vi "Processed_Bytes_To_Data_Packet.vi"(2 "Processed Bytes":u8[](array[numeric]), 3 "Data Packet In":T1) -> (1 "Data Packet Out":T1)   [LabVIEW 2017]
uses:
  Controls/Packet/Packet.ctl
  Controls/Packet/Packet_Direction.ctl
  Controls/Packet/Packet_Type.ctl
  Controls/Packet/Packet_Priority.ctl
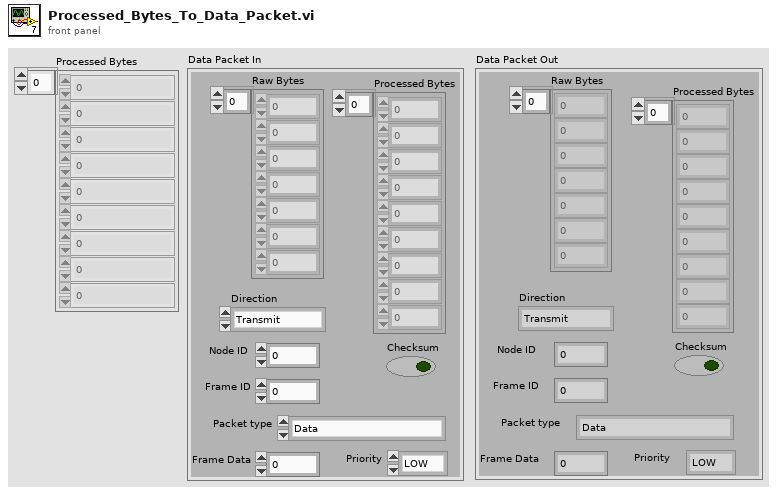
[diagram p1: front panel]
types:
  T1 = typedef "Packet.ctl" = cluster{"Raw Bytes":u8[], "Checksum":bool, "Direction":T2, "Processed Bytes":u8[], "Node ID":u8, "Packet type":T3, "Frame Data":u32, "Priority":T4, "Frame ID":u8}
  T2 = typedef "Packet_Direction.ctl" = enum16{"Transmit", "Receive", "Bidirectional"}
  T3 = typedef "Packet_Type.ctl" = enum16{"Data", "Connection Management", "Remote Request", "Error/Status"}
  T4 = typedef "Packet_Priority.ctl" = enum16{"LOW", "HIGH"}
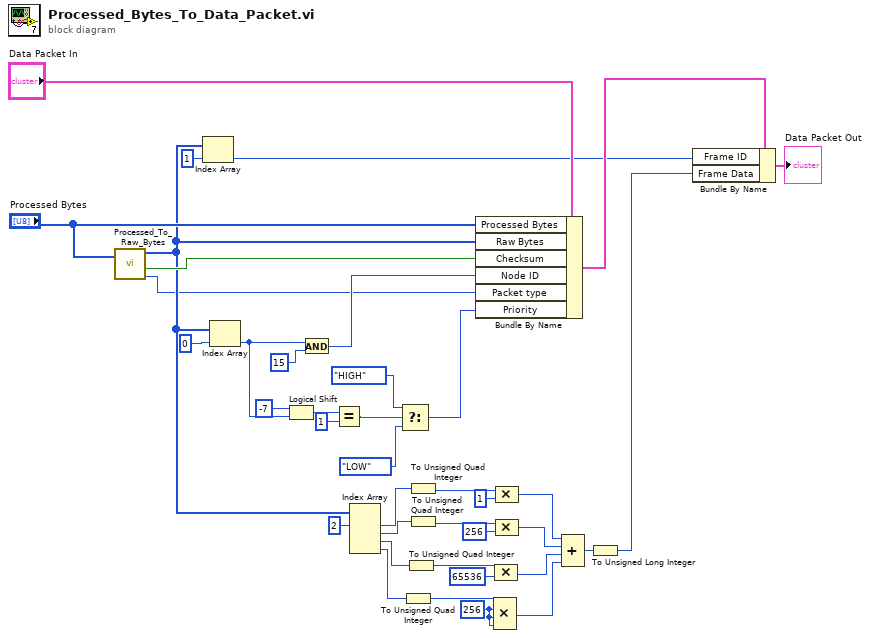
[diagram p0: block diagram]
diagram:
  w9 = u64 256 ("value")
  n1 = call "Processed_To_Raw_Bytes.vi"("Processed Bytes"="Processed Bytes") -> ("Packet Type"=w1:T3, "Checksum"=w37:bool, "Raw Bytes"=w22:u8[])  [unwired: 1 in, 2 out]
  n2 = Index Array(array=w22, index=1) -> (element=w23:u8)
  n3 = Index Array(array=w22, index=0) -> (element=w33:u8)
  n4 = Logical Shift(y=i16 -7, x=w33) -> (x << y=w31:u8)
  n5 = And(x=w33, y=u8 15) -> (x .and. y?=w34:u8)
  n6 = Equal?(x=w31, y=u8 1) -> (x = y?=w29:bool)
  n7 = Index Array(array=w22, index #1=2 ("index")) -> (element #1=w20:u8, element #2=w19:u8, element #3=w18:u8, element #4=w17:u8)  [unwired: 3 in]
  n8 = Select(t=Packet_Priority."HIGH" ("Enum"), s=w29, f=Packet_Priority."LOW") -> (s? t:f=w26:T4)
  n9 = To Unsigned Quad Integer(1:w17) -> (0:w10:u64)
  n10 = To Unsigned Quad Integer(1:w18) -> (0:w12:u64)
  n11 = To Unsigned Quad Integer(1:w20) -> (0:w16:u64)
  n12 = To Unsigned Quad Integer(1:w19) -> (0:w14:u64)
  n13 = Bundle By Name(cluster="Data Packet In", "Processed Bytes"="Processed Bytes", "Raw Bytes"=w22, "Checksum"=w37, "Node ID"=w34, "Packet type"=w1, "Priority"=w26) -> (w25:T1)
  n14 = Compound Arithmetic op=MULTIPLY(w10, w9, w9, w9) -> (w5:u64)
  n15 = Compound Arithmetic op=MULTIPLY(w12, u64 65536 ("value")) -> (w6:u64)
  n16 = Compound Arithmetic op=MULTIPLY(w16, u64 1 ("value")) -> (w8:u64)
  n17 = Compound Arithmetic op=MULTIPLY(w14, u64 256 ("value")) -> (w7:u64)
  n18 = Compound Arithmetic op=ADD(w8, w7, w6, w5) -> (w4:u64)
  n19 = To Unsigned Long Integer(number=w4) -> (unsigned 32bit integer=w3:u32)
  n20 = Bundle By Name(cluster=w25, "Frame ID"=w23, "Frame Data"=w3) -> (→"Data Packet Out":T1)
